vi "MotionState.vi"(8 "Error In":errorcluster, 9 "等候秒數":i32=100, 10 "index":i32=15, 11 "IP:Port":string) -> (0 "error out":errorcluster, 1 "Error status":bool, 2 "移動完成":bool, 3 "Motion State":bool[](array[boolean]), 4 "等候逾時":bool, 5 "剩餘秒數":i32)   [LabVIEW 2019, in "Kolmogan Library 1.lvlib"]
uses:
  Kolmogan Library 1.lvlib
panel:
  # "一秒\n大約五十秒"
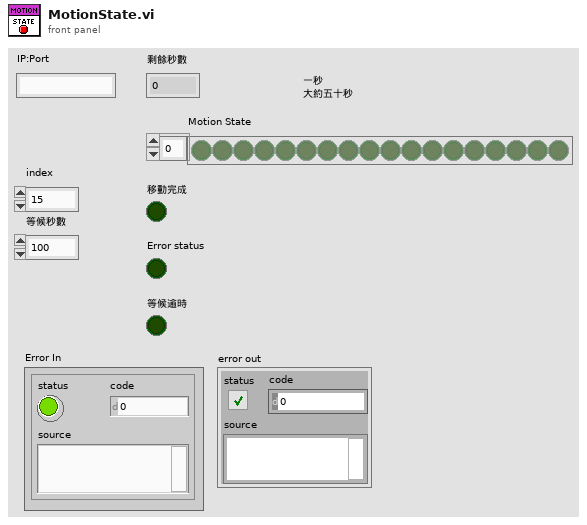
[diagram p1: front panel]
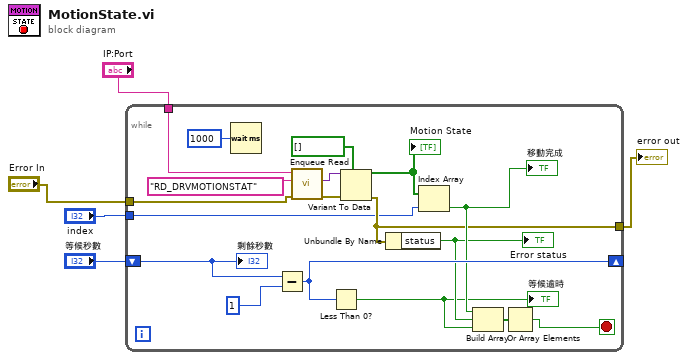
[diagram p0: block diagram]
diagram:
  n1 = while {
    tunnel: "IP:Port" -> [w19]
    shift-right: [w15] -> _
    shift-left: "等候秒數" -> [w17]
    tunnel: [w8] -> w5
    tunnel: "index" -> [w7]
    tunnel: "Error In" -> [w6]
    stop <- w10 stop-if-true
    n2 = Wait (ms)(milliseconds to wait=u32 1000) -> ()  [unwired: 1 out]
    n3 = Subtract(x=w17, y=1) -> (x-y=w15:i32)
    n4 = call "Enqueue Read.vi"("Error In"=w6, "Message"="RD_DRVMOTIONSTAT", "Name"=w19) -> ("Error Out"=w23:errorcluster, "Data"=w22:variant)  [unwired: 7 in]
    n5 = Less Than 0?(x=w15) -> (x < 0?=w12:bool)
    "等候逾時" <- w12
    n6 = Variant To Data(error in=w23, type=bool[] [] ("appended array"), Variant=w22) -> (data=w18:bool[], error out=w8:errorcluster)
    "Motion State" <- w18
    n7 = Unbundle By Name(w8) -> ("status"=w13:bool)
    "Error status" <- w13
    n8 = Index Array(array=w18, index=w7) -> (element=w14:bool)
    "移動完成" <- w14
    n9 = Build Array(w14, w13, w12) -> (w11:bool[])
    n10 = Or Array Elements(Boolean array=w11) -> (logical OR=w10:bool)
    "剩餘秒數" <- w17
  }
  "error out" <- w5
